vi "Sample_EL72xx_MotionControl.vi"() -> ()   [LabVIEW 2022 SP3, in "Motion_Library.lvlib"]
uses:
  Motion_Library.lvlib
  TypeDefs/EL72xx_DMCInputs.ctl
  TypeDefs/EL72xx_DMCOutputs.ctl
  ADS/ADS_Library.lvlib
panel:
  out "bHasMatched":bool
  out "Write Status":bool
  in  "DMC Outputs":T1
  out "data":T2
  out "Read status?":bool
  in  "stop":bool
  in  "PortInfo":string="<PortInfo><Inputs><SymbolControlItems><SymbolControlItem GroupName=\"ADS Write\" GroupDescription=\"Parameters for ADS Write command\"><Parameters><Parameter Name=\"Name\">Term 27 (EL7201-9014).DMC Outputs 32 Bit</Parameter><Parameter Name=\"SymbolName\">Term 27 (EL7201-9014).DMC Outputs 32 Bit</Parameter><Parameter Name=\"SymbolType\">DMC Outputs 32 Bit_TYPE</Parameter><Parameter Name=\"SymbolGuid\"></Parameter><Parameter Name=\"AmsNetId\">192.168.80.50.1.1</Parameter><Parameter Name=\"Port\">27906</Parameter><Parameter Name=\"IndexGroup\">#x0</Parameter><Parameter Name=\"IndexOffset\">#x0</Parameter><Parameter Name=\"BitSize\">320</Parameter><Parameter Name=\"CycleTime [ms]\">10</Parameter><Parameter Name=\"Timeout [ms]\">1000</Parameter></Parameters></SymbolControlItem></SymbolControlItems></Inputs><Outputs><SymbolControlItems><SymbolControlItem GroupName=\"ADS Read\" GroupDescription=\"Parameters for ADS Read command\"><Parameters><Parameter Name=\"Name\">Term 27 (EL7201-9014).DMC Inputs 32 Bit</Parameter><Parameter Name=\"SymbolName\">Term 27 (EL7201-9014).DMC Inputs 32 Bit</Parameter><Parameter Name=\"SymbolType\">DMC Inputs 32 Bit_TYPE</Parameter><Parameter Name=\"SymbolGuid\"></Parameter><Parameter Name=\"AmsNetId\">192.168.80.50.1.1</Parameter><Parameter Name=\"Port\">27906</Parameter><Parameter Name=\"IndexGroup\">#x0</Parameter><Parameter Name=\"IndexOffset\">#x0</Parameter><Parameter Name=\"BitSize\">512</Parameter><Parameter Name=\"CycleTime [ms]\">10</Parameter><Parameter Name=\"Transmode\">3</Parameter><Parameter Name=\"Timeout [ms]\">1000</Parameter><Parameter Name=\"TCBufferSize [Samples]\">10</Parameter><Parameter Name=\"LVBufferSize [Samples]\">50</Parameter><Parameter Name=\"Expected min delay [ms]\">500</Parameter></Parameters></SymbolControlItem></SymbolControlItems></Outputs></PortInfo>"
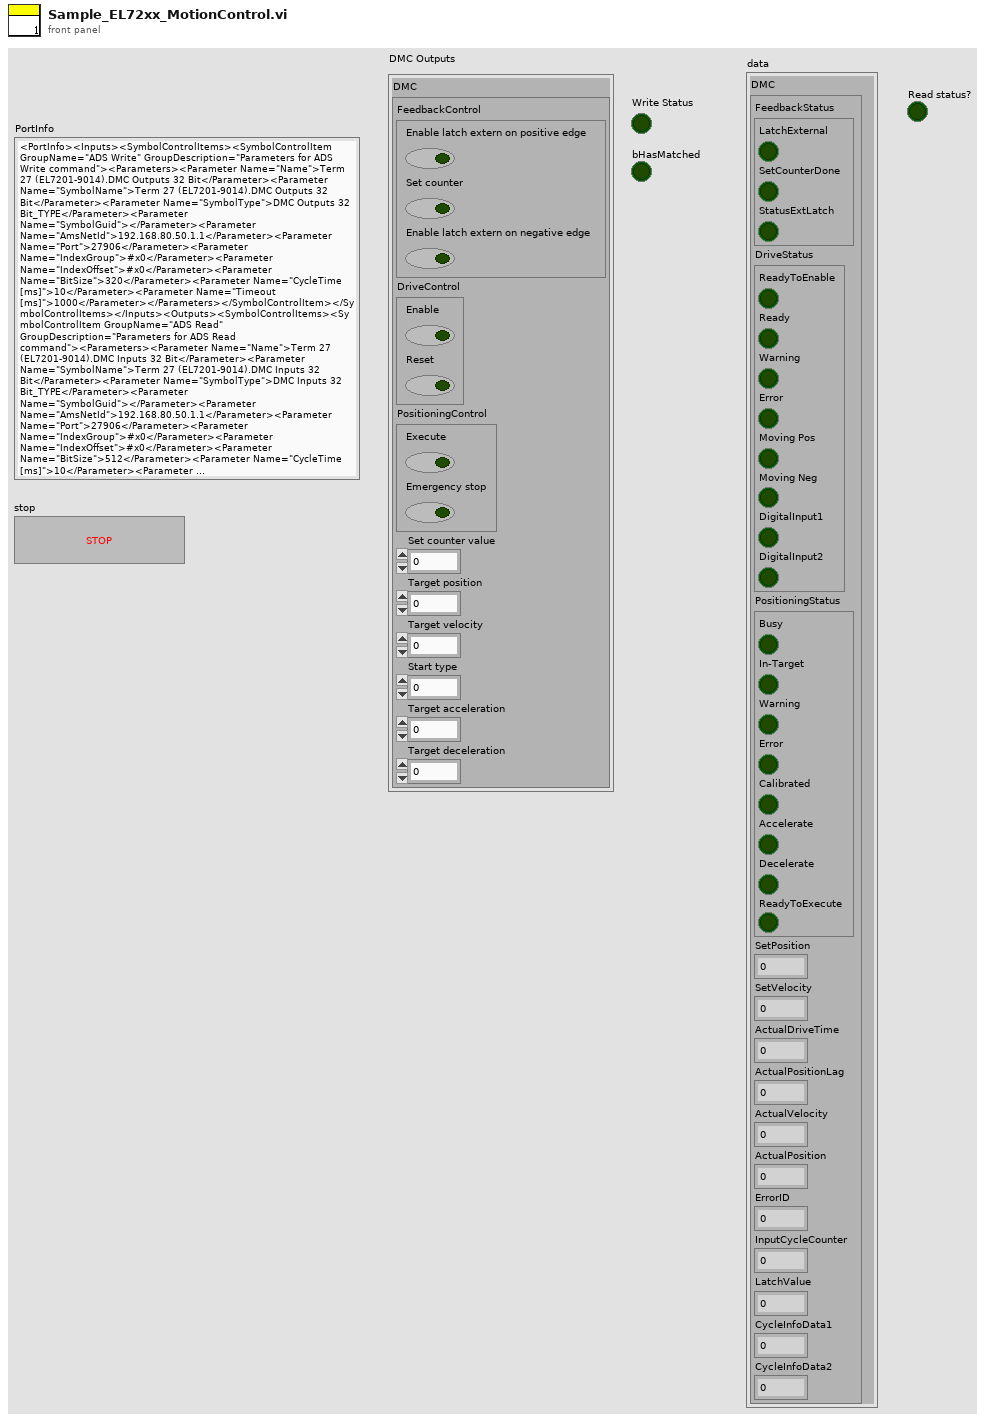
[diagram p1: front panel]
types:
  T1 = typedef "Motion_Library.lvlib/EL72xx_DMCOutputs.ctl" = cluster{"DMC":cluster{"FeedbackControl":cluster{"Enable latch extern on positive edge":bool, "Set counter":bool, "Enable latch extern on negative edge":bool}, "DriveControl":cluster{"Enable":bool, "Reset":bool}, "PositioningControl":cluster{"Execute":bool, "Emergency stop":bool}, "Set counter value":i32, "Target position":i32, "Target velocity":i16, "Start type":u16, "Target acceleration":u16, "Target deceleration":u16}}
  T2 = typedef "Motion_Library.lvlib/EL72xx_DMCInputs.ctl" = cluster{"DMC":cluster{"FeedbackStatus":cluster{"LatchExternal":bool, "SetCounterDone":bool, "StatusExtLatch":bool}, "DriveStatus":cluster{"ReadyToEnable":bool, "Ready":bool, "Warning":bool, "Error":bool, "Moving Pos":bool, "Moving Neg":bool, "DigitalInput1":bool, "DigitalInput2":bool}, "PositioningStatus":cluster{"Busy":bool, "In-Target":bool, "Warning":bool, "Error":bool, "Calibrated":bool, "Accelerate":bool, "Decelerate":bool, "ReadyToExecute":bool}, "SetPosition":dbl, "SetVelocity":dbl, "ActualDriveTime":dbl, "ActualPositionLag":dbl, "ActualVelocity":dbl, "ActualPosition":dbl, "ErrorID":dbl, "InputCycleCounter":dbl, "LatchValue":dbl, "CycleInfoData1":dbl, "CycleInfoData2":dbl}}
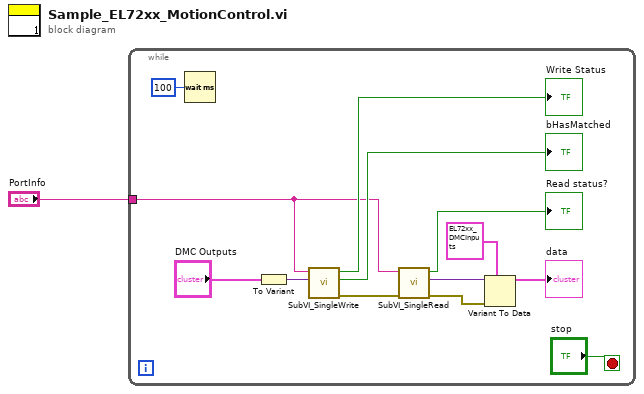
[diagram p0: block diagram]
diagram:
  n1 = while {
    tunnel: "PortInfo" -> [w2]
    stop <- "stop" stop-if-true
    n2 = Wait (ms)(milliseconds to wait=u32 100) -> ()  [unwired: 1 out]
    n3 = To Variant(anything="DMC Outputs") -> (Variant=w6:variant)
    n4 = call "SubVI_SingleWrite.vi"("WData"=w6, "String"=w2) -> ("error out"=w5:errorcluster, "bHasMatched"=→"bHasMatched":bool, "Write Status"=→"Write Status":bool)  [unwired: 6 in, 1 out]
    n5 = call "SubVI_SingleRead.vi"("error in"=w5, "String"=w2) -> ("error out"=w11:errorcluster, "RData"=w12:variant, "Read status?"=→"Read status?":bool)  [unwired: 6 in]
    n6 = Variant To Data(error in=w11, type=T2 {"DMC"={"FeedbackStatus"={"LatchExternal"=FALSE, "SetCounterDone"=FALSE, "StatusExtLatch"=FALSE}, "DriveStatus"={"ReadyToEnable"=FALSE, "Ready"=FALSE, "Warning"=FALSE, "Error"=FALSE, "Moving Pos"=FALSE, "Moving Neg"=FALSE, "DigitalInput1"=FALSE, "DigitalInput2"=FALSE}, "PositioningStatus"={"Busy"=FALSE, "In-Target"=FALSE, "Warning"=FALSE, "Error"=FALSE, "Calibrated"=FALSE, "Accelerate"=FALSE, "Decelerate"=FALSE, "ReadyToExecute"=FALSE}, "SetPosition"=0.0, "SetVelocity"=0.0, "ActualDriveTime"=0.0, "ActualPositionLag"=0.0, "ActualVelocity"=0.0, "ActualPosition"=0.0, "ErrorID"=0.0, "InputCycleCounter"=0.0, "LatchValue"=0.0, "CycleInfoData1"=0.0, "CycleInfoData2"=0.0}} ("DMC Inputs"), Variant=w12) -> (data=→"data":T2)  [unwired: 1 out]
  }
